vi "Drive Controller.vi"(8 "error in":errorcluster) -> ()   [LabVIEW 2020]
doc: "This VI executes continuously carrying out the current operation and responding to updates or new operation requests. It will often contain the timing or control code that is difficult to place directly in TeleOp. This VI generally opens all sensors and motors and isolates the rest of the robot code from knowing implementation details of how the operations are carried out."
uses:
  <vilib>/Rock Robotics/WPI/Framework/Completion Status.ctl
  Drive Setpoints.ctl
  Drive Operations.ctl
  <vilib>/Rock Robotics/WPI/SafetyOutput/WPI_SafetyOutputConfigMenu.ctl
  <vilib>/Rock Robotics/WPI/RobotDrive/WPI_RobotDriveOpen2MotorWithExistingMotors.vi
  <vilib>/Rock Robotics/Network Tables/NT Write Numeric Array.vi
panel:
  in  "Interactive Values":T1
  in  "Buttons":cluster{"Execute Cmd":bool, "Abort Cmd":bool}
  out "Command Timing":cluster{"Start Time (ms)":u32, "Iterations":i32}
  out "Status":T3
  out "Setpoints":T4(graph)
  out "Current\nCmd":string
  # "Tip: The graph shows the motor setpoints. It may also be helpful to observe inputs and sensor values.\nYou may also want to display tuning or debugging controls."
  # "Interactive Command: You may fill in the settings for a command\nand schedule it with the Execute button. You can observe and abort\nany command while fine tuning the code for the controller."
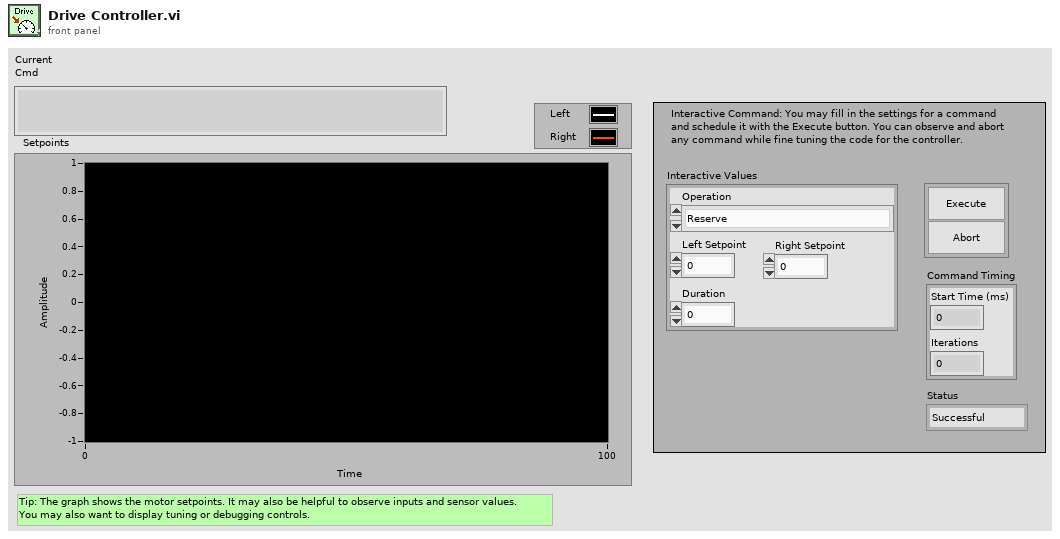
[diagram p1: front panel]
types:
  T1 = typedef "Drive Setpoints.ctl" = cluster{"Operation":T2, "Left Setpoint":dbl, "Right Setpoint":dbl, "Duration":dbl}
  T2 = typedef "Drive Operations.ctl" = enum16{"Reserve", "Read Current", "Immediate", "Drive for Time", "Drive for Distance"}
  T3 = typedef "Completion Status.ctl" = enum16{"Successful", "Aborted", "Incomplete"}
  T4 = cluster{"Left Setpoint":dbl, "Right Setpoint":dbl}
  T5 = typedef "WPI_SafetyOutputConfigMenu.ctl" = enum16{"Enable", "Disable"}
  T6 = typedef "WPI_MotorControlDeviceRef.ctl" = cluster{"DeviceStatus":errorcluster, "Type":T7, "PWM":cluster{"PWM Channel":T8, "DeadBand":T9}, "CAN":cluster{"Device Number":u8, "SetOutput VI Ref":variant, "GetOutput VI Ref":variant, "Enable VI Ref":variant, "Disable VI Ref":variant, "Data":variant}, "Invert":bool, "DIO PWM":cluster{"PWM \"Enable\" Channel":T8, "DIOChannel":T10, "PWM Rate":dbl}}
  T7 = typedef "WPI_MotorControlType.ctl" = enum16{"PWM", "CAN", "DIO PWM"}
  T8 = typedef "FPGA_DIOPWMChannel.ctl" = enum8{"PWM 0", "PWM 1", "PWM 2", "PWM 3", "PWM 4", "PWM 5", "PWM 6", "PWM 7", "PWM 8", "PWM 9", "PWM MXP 0", "PWM MXP 1", "PWM MXP 2", "PWM MXP 3", "PWM MXP 4", "PWM MXP 5", "PWM MXP 6", "PWM MXP 7", "PWM MXP 8", "PWM MXP 9", "Invalid"}
  T9 = typedef "WPI_PWMDeadband.ctl" = cluster{"Name":string, "maxPositivePwm":i32, "minPositivePwm":i32, "centerPwm":i32, "maxNegativePwm":i32, "minNegativePwm":i32, "angularRange":u16}
  T10 = typedef "FPGA_DIOChannel.ctl" = enum8{"DIO 0", "DIO 1", "DIO 2", "DIO 3", "DIO 4", "DIO 5", "DIO 6", "DIO 7", "DIO 8", "DIO 9", "DIO MXP 0", "DIO MXP 1", "DIO MXP 2", "DIO MXP 3", "DIO MXP 4", "DIO MXP 5", "DIO MXP 6", "DIO MXP 7", "DIO MXP 8", "DIO MXP 9", "DIO MXP 10", "DIO MXP 11", "DIO MXP 12", "DIO MXP 13", "DIO MXP 14", "DIO MXP 15", "SPI Port CS1", "SPI Port CS2", "SPI Port CS3", "SPI Port MISO", "SPI Port MOSI", "Invalid"}
  T11 = typedef "WPI_RobotDriveDevRef.ctl" = cluster{"DevStatus":errorcluster, "Motors[]":T6[], "Square Inputs":bool, "Max Output":dbl}
  T12 = typedef "Command Status Info.ctl" = cluster{"Name":string, "Status":T3, "notifier out":T13}
  T13 = typedef "Completion Notifier.ctl" = refnum<notifier>
  T14 = cluster{"SubSystem Data":T1, cluster{"Start Time (ms)":u32, "Iterations":i32}, cluster{"Command Info":T12, "Description":string, "Default Command":T1, "queue out":refnum<queue>, "Subsystem Name":string}}
  T15 = cluster{"SubSystem Data":T1, cluster{"Start Time (ms)":u32, "Iterations":i32}, "Default Command Arguments":cluster{"Command Info":T12, "Description":string, "Default Command":T1, "queue out":refnum<queue>, "Subsystem Name":string}}
  T16 = cluster{"Don't move motors while reserved":dbl, "Don't move motors while reserved":dbl}
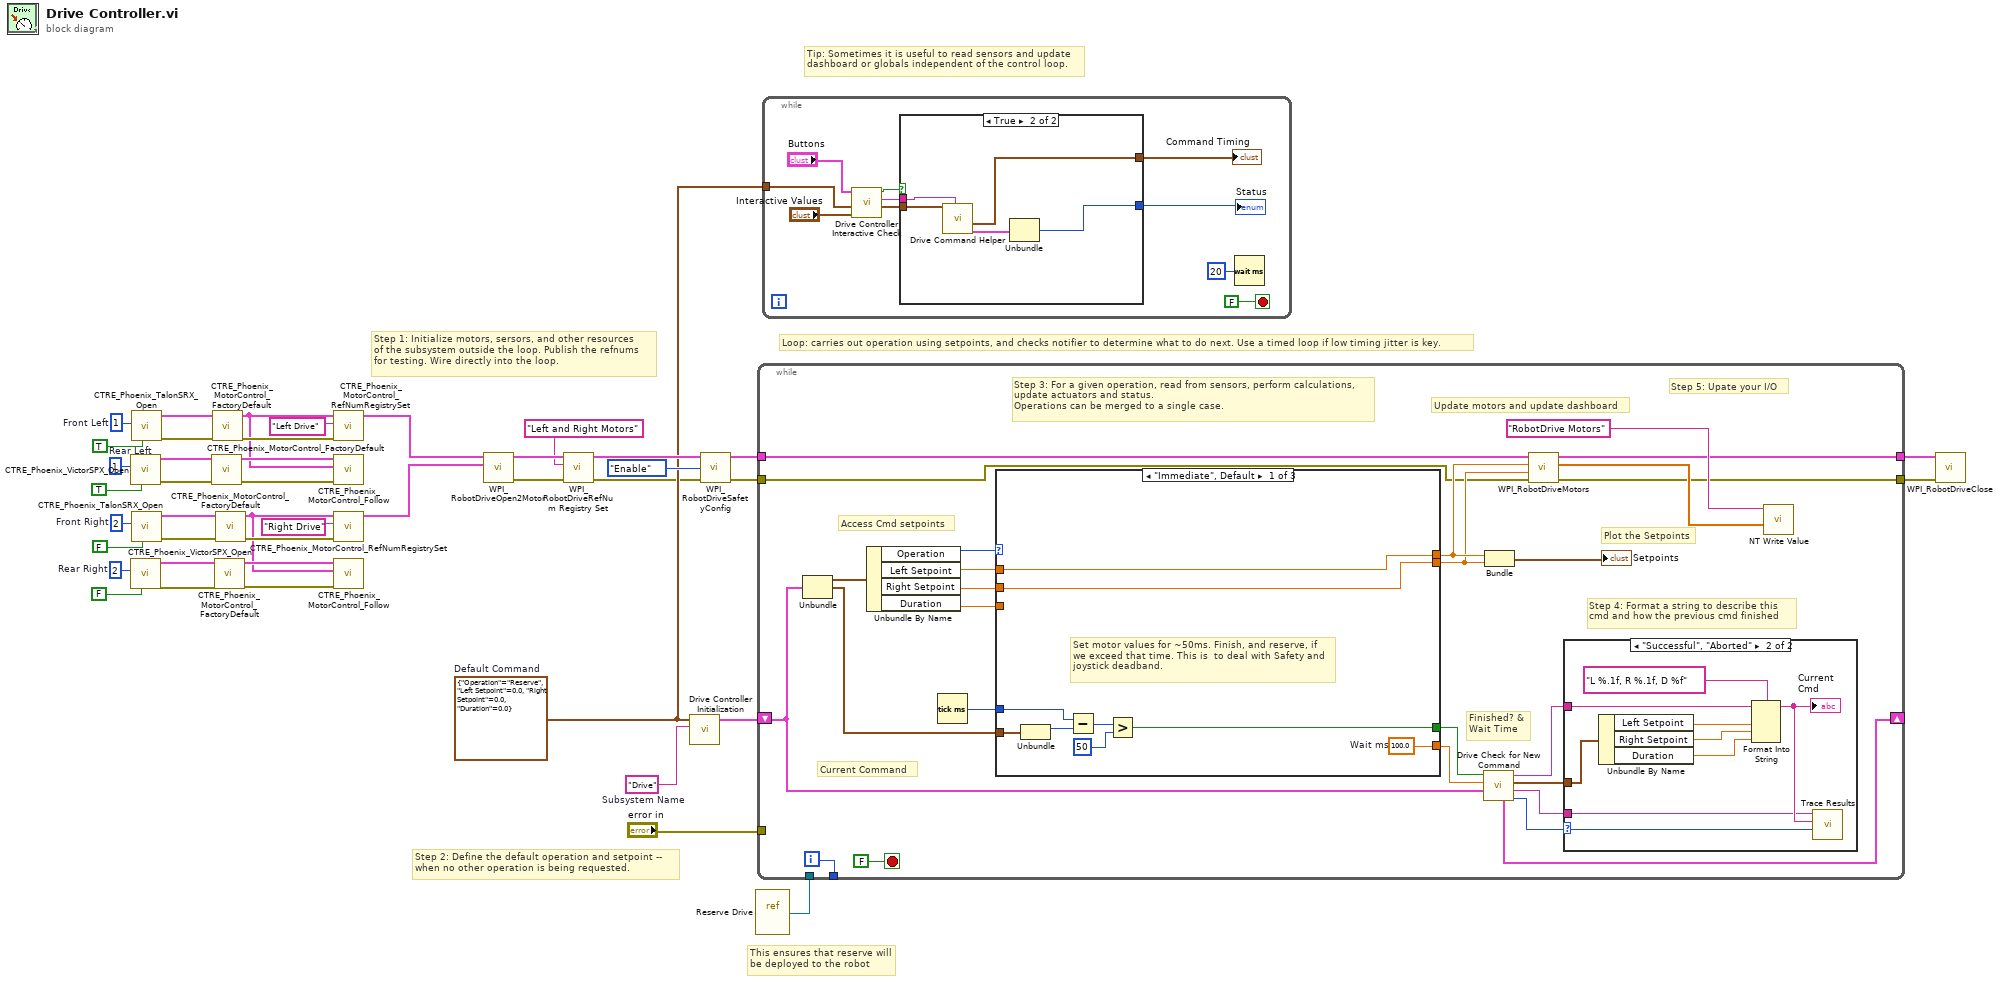
[diagram p0: block diagram]
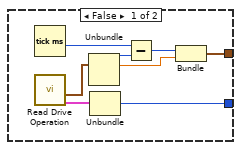
[diagram p2: hidden frame]
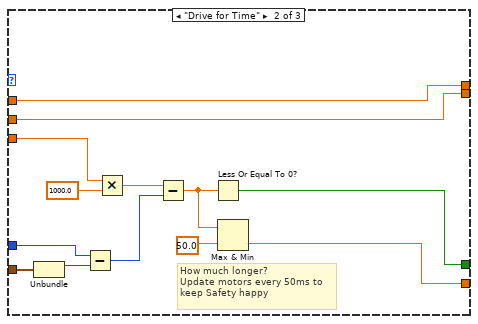
[diagram p4: hidden frame]
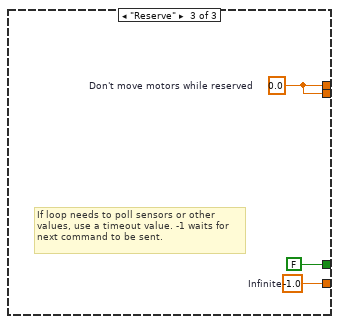
[diagram p5: hidden frame]
diagram:
  w11 = u8 2  # Front Right
  w12 = u8 2  # Rear Right
  w13 = u8 1  # Front Left
  w14 = u8 1  # Rear Left
  w33 = T1 {"Operation"=enum."Reserve", "Left Setpoint"=0.0, "Right Setpoint"=0.0, "Duration"=0.0}  # Default Command
  w43 = "Drive"  # Subsystem Name
  # "This ensures that reserve will\nbe deployed to the robot"
  # "Tip: Sometimes it is useful to read sensors and update\ndashboard or globals independent of the control loop."
  # "Step 2: Define the default operation and setpoint --\nwhen no other operation is being requested."
  # "Step 1: Initialize motors, sersors, and other resources\nof the subsystem outside the loop. Publish the refnums\nfor testing. Wire directly into the loop."
  # "Loop: carries out operation using setpoints, and checks notifier to determine what to do next. Use a timed loop if low timing jitter is key."
  n1 = call <vilib>:"CTRE_Phoenix_VictorSPX_Open.vi"("Invert"=TRUE, "Device Number"=w14) -> ("error out"=w32:errorcluster, "PhoenixMotorControlDevRef"=w31:T6)  [unwired: 8 in]
  n2 = call <vilib>:"CTRE_Phoenix_VictorSPX_Open.vi"("Invert"=FALSE, "Device Number"=w12) -> ("error out"=w29:errorcluster, "PhoenixMotorControlDevRef"=w30:T6)  [unwired: 8 in]
  n3 = call <vilib>:"CTRE_Phoenix_TalonSRX_Open.vi"("Invert"=TRUE, "Device Number"=w13) -> ("error out"=w24:errorcluster, "PhoenixMotorControlDevRef"=w23:T6)  [unwired: 8 in]
  n4 = call <vilib>:"CTRE_Phoenix_TalonSRX_Open.vi"("Invert"=FALSE, "Device Number"=w11) -> ("error out"=w22:errorcluster, "PhoenixMotorControlDevRef"=w21:T6)  [unwired: 8 in]
  n5 = call <vilib>:"CTRE_Phoenix_MotorControl_FactoryDefault.vi"("error in"=w32, "PhoenixMotorControlDevRef"=w31) -> ("error out"=w26:errorcluster, "PhoenixMotorControlDevRef"=w25:T6)  [unwired: 8 in]
  n6 = call <vilib>:"CTRE_Phoenix_MotorControl_FactoryDefault.vi"("error in"=w24, "PhoenixMotorControlDevRef"=w23) -> ("error out"=w18:errorcluster, "PhoenixMotorControlDevRef"=w17:T6)  [unwired: 8 in]
  n7 = call <vilib>:"CTRE_Phoenix_MotorControl_FactoryDefault.vi"("error in"=w29, "PhoenixMotorControlDevRef"=w30) -> ("error out"=w28:errorcluster, "PhoenixMotorControlDevRef"=w27:T6)  [unwired: 8 in]
  n8 = call <vilib>:"CTRE_Phoenix_MotorControl_FactoryDefault.vi"("error in"=w22, "PhoenixMotorControlDevRef"=w21) -> ("error out"=w20:errorcluster, "PhoenixMotorControlDevRef"=w19:T6)  [unwired: 8 in]
  n9 = call <vilib>:"CTRE_Phoenix_MotorControl_RefNumRegistrySet.vi"("error in (no error)"=w18, "refnum name"="Left Drive", "PhoenixMotorControlDevRef"=w17) -> ("PhoenixMotorControlDevRef"=w10:T6)  [unwired: 7 in, 1 out]
  n10 = call <vilib>:"CTRE_Phoenix_MotorControl_Follow.vi"("error in (no error)"=w26, "Master Controller to Follow"=w17, "PhoenixMotorControlDevRef"=w25) -> ()  [unwired: 7 in, 2 out]
  n11 = call <vilib>:"CTRE_Phoenix_MotorControl_RefNumRegistrySet.vi"("error in (no error)"=w20, "refnum name"="Right Drive", "PhoenixMotorControlDevRef"=w19) -> ("PhoenixMotorControlDevRef"=w9:T6)  [unwired: 7 in, 1 out]
  n12 = call <vilib>:"CTRE_Phoenix_MotorControl_Follow.vi"("error in (no error)"=w28, "Master Controller to Follow"=w19, "PhoenixMotorControlDevRef"=w27) -> ()  [unwired: 7 in, 2 out]
  n13 = call-poly <vilib>:"WPI_RobotDriveOpen2Motor.vi"("Right Motor Dev Ref"=w9, "Left Motor Dev Ref"=w10) -> ("error out"=w40:errorcluster, "RobotDriveDevRef"=w42:T11)  [unwired: 3 in, 5 out]
  n14 = call <vilib>:"WPI_RobotDriveRefNum Registry Set.vi"("error in (no error)"=w40, "refnum name"="Left and Right Motors", "RobotDriveDevRef"=w42) -> ("error out"=w3:errorcluster, "RobotDriveDevRef"=w39:T11)  [unwired: 1 in, 6 out]
  n15 = call "Drive Controller Initialization.vi"("Subsystem Name"=w43, "Default Command"=w33) -> ("Current Command"=w35:T14)  [unwired: 9 in]
  n16 = call <vilib>:"WPI_RobotDriveSafetyConfig.vi"("error in (no error)"=w3, "mode"=WPI_SafetyOutputConfigMenu."Enable", "RobotDriveDevRef"=w39) -> ("error out"=w2:errorcluster, "RobotDriveDevRef"=w37:T11)  [unwired: 7 in]
  n17 = vi-ref "Reserve Drive.vi"() -> (w34:refnum<vi>)
  n18 = while {
    shift-right: [w56] -> _
    shift-left: w35 -> [w49]
    tunnel: [w68] -> _
    tunnel: w37 -> [w64]
    tunnel: "error in" -> [_]
    tunnel: w34 -> [_]
    tunnel: [w46] -> w8
    tunnel: w2 -> [w45]
    tunnel: [w44] -> w1
    i -> [w68]
    stop <- FALSE stop-if-true
    # "Step 5: Upate your I/O"
    # "Step 4: Format a string to describe this\ncmd and how the previous cmd finished"
    # "Current Command"
    # "Update motors and update dashboard"
    # "Plot the Setpoints"
    # "Access Cmd setpoints"
    # "Finished? &\nWait Time"
    # "Step 3: For a given operation, read from sensors, perform calculations,\nupdate actuators and status.\nOperations can be merged to a single case."
    n19 = Unbundle(w49) -> ("SubSystem Data"=w63:T1, w50:cluster{"Start Time (ms)":u32, "Iterations":i32})  [unwired: 1 out]
    n20 = Unbundle By Name(w63) -> ("Operation"=w62:T2, "Left Setpoint"=w61:dbl, "Right Setpoint"=w60:dbl, "Duration"=w59:dbl)
    n21 = Tick Count (ms)() -> (millisecond timer value=w58:u32)
    n22 = case shown="\"Immediate\", Default" w62 {
      tunnel: [w87 w88 w103] -> w55
      tunnel: [w80 w95 FALSE ("ignore previous (F)")] -> w54
      tunnel: w50 -> [w79 w97 _]
      tunnel: [w86 w94 w101] -> w66
      tunnel: [w85 w93 w101] -> w65
      tunnel: w61 -> [w86 w94 _]
      tunnel: w60 -> [w85 w93 _]
      tunnel: w59 -> [_ w92 _]
      tunnel: w58 -> [w81 w91 _]
      frame "Immediate", Default {
        w87 = 100.0  # Wait ms
        # "Set motor values for ~50ms. Finish, and reserve, if\nwe exceed that time. This is  to deal with Safety and\njoystick deadband."
        n23 = Unbundle(w79) -> ("Start Time (ms)"=w82:u32)  [unwired: 1 out]
        n24 = Subtract(x=w81, y=w82) -> (x-y=w83:u32)
        n25 = Greater?(x=w83, y=u8 50 ("Left Motor")) -> (0:w80:bool)
      }
      frame "Drive for Time" {
        # "How much longer?\nUpdate motors every 50ms to\nkeep Safety happy"
        n26 = Unbundle(w97) -> ("Start Time (ms)"=w96:u32)  [unwired: 1 out]
        n27 = Subtract(x=w91, y=w96) -> (x-y=w100:u32)
        n28 = Multiply(x=w92, y=1000.0) -> (x*y=w99:dbl)
        n29 = Subtract(x=w99, y=w100) -> (x-y=w90:dbl)
        n30 = Less Or Equal To 0?(x=w90) -> (x <= 0?=w95:bool)
        n31 = Max & Min(x=w90, y=50.0) -> (min(x,y)=w88:dbl)  [unwired: 1 out]
      }
      frame "Reserve" {
        w101 = 0.0  # Don't move motors while reserved
        w103 = -1.0  # Infinite
        # "If loop needs to poll sensors or other\nvalues, use a timeout value. -1 waits for\nnext command to be sent."
      }
    }
    n32 = call "Drive Check for New Command.vi"("input cluster"=w49, "Wait time (ms)"=w55, "Finished?"=w54) -> ("Completion"=w57:T3, "Subsystem Name"=w51:string, "Current Command"=w52:T1, "Initial Trace String"=w53:string, "Next Command"=w56:T15)  [unwired: 4 in]
    n33 = Bundle("Don't move motors while reserved"=w66, "Don't move motors while reserved"=w65) -> (→"Setpoints":T16)  [unwired: 1 in]
    n34 = call <vilib>:"WPI_RobotDriveMotors.vi"("error in (no error)"=w45, "RightSpeed"=w65, "LeftSpeed"=w66, "RobotDriveDevRef"=w64) -> ("error out"=w44:errorcluster, "Motor Values"=w47:dbl[], "RobotDriveDevRef"=w46:T11)  [unwired: 5 out]
    n35 = case shown="\"Successful\", \"Aborted\"" w57 {
      selector: w57 -> [_ w78]
      tunnel: w53 -> [_ w73]
      tunnel: w52 -> [_ w74]
      tunnel: w51 -> [_ w70]
      frame "Incomplete", Default {
        # "Continuing current command"
      }
      frame "Successful", "Aborted" {
        # "Report and setup for next command"
        n36 = Unbundle By Name(w74) -> ("Left Setpoint"=w76:dbl, "Right Setpoint"=w77:dbl, "Duration"=w71:dbl)
        n37 = Format Into String(format string="L %.1f, R %.1f, D %f", initial string=w73, w76, w77, w71) -> (resulting string=w72:string)  [unwired: 1 in, 1 out]
        "Current\nCmd" <- w72
        n38 = call <vilib>:"Trace Results.vi"("Status of previous command"=w78, "Description"=w72, "Subsystem"=w70) -> ()  [unwired: 9 in]
      }
    }
    n39 = call-poly <vilib>:"NT Write Value.vi"("Numeric Array"=w47, "Name"="RobotDrive Motors") -> ()  [unwired: 9 in, 1 out]
  }
  n40 = while {
    tunnel: w33 -> [w105]
    stop <- FALSE stop-if-true
    n41 = call "Drive Controller Interactive Check.vi"("Interactive Command In"="Interactive Values", "Default Command"=w105, "Buttons"="Buttons") -> ("Interactive Command Out"=w107:T1, "Trace String"=w108:string, "Schedule"=w109:bool)  [unwired: 6 in]
    n42 = case shown="True" w109 {
      tunnel: [w118 w126] -> w110
      tunnel: [w117 w122] -> w111
      tunnel: w108 -> [_ w124]
      tunnel: w107 -> [_ w123]
      frame False {
        n43 = Tick Count (ms)() -> (millisecond timer value=w121:u32)
        n44 = call "Read Drive Operation.vi"() -> ("Command Info"=w115:T12, "SubSystem Data"=w114:T1)  [unwired: 9 in, 1 out]
        n45 = Unbundle(w114) -> ("Operation"=w119:T2, "Left Setpoint"=w116:dbl)  [unwired: 2 out]
        n46 = Unbundle(w115) -> ("Status"=w118:T3)  [unwired: 2 out]
        n47 = Subtract(x=w121, y=w119) -> (x-y=w120:u32)
        n48 = Bundle(w120, "Left Setpoint"=w116) -> (w117:cluster{u32, "Left Setpoint":dbl})  [unwired: 1 in]
      }
      frame True {
        n49 = call "Drive Command Helper.vi"("Description"=w124, "SubSystem Data"=w123) -> ("Command Info Out"=w125:T12, "Command Timing"=w122:cluster{"Start Time (ms)":u32, "Iterations":i32})  [unwired: 7 in, 1 out]
        n50 = Unbundle(w125) -> ("Status"=w126:T3)  [unwired: 2 out]
      }
    }
    "Status" <- w110
    "Command Timing" <- w111
    n51 = Wait (ms)(milliseconds to wait=u32 20) -> ()  [unwired: 1 out]
  }
  n52 = call <vilib>:"WPI_RobotDriveClose.vi"("error in (no error)"=w1, "RobotDriveDevRef"=w8) -> ()  [unwired: 9 in, 1 out]
